vi "SLM Save Frame 640.vi"(4 "Pixel Values":u8[](array[numeric]), 5 "error in (no error)":errorcluster, 6 "Frame Number":u32, 7 "Number of Pixels":u32, 8 "VISA Resource Name":refnum<visa-resource-name>) -> (0 "error out":errorcluster, 3 "dup VISA resource name":refnum<visa-resource-name>)   [LabVIEW 2022 SP3]
panel:
  out "num pixels":u32(graph)
  out "size(s)":i32(graph)
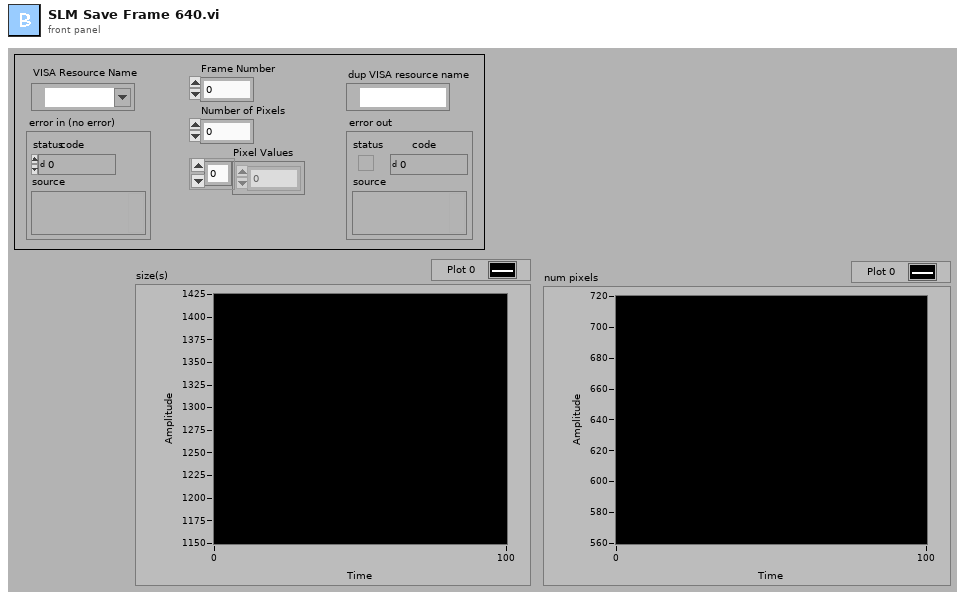
[diagram p1: front panel]
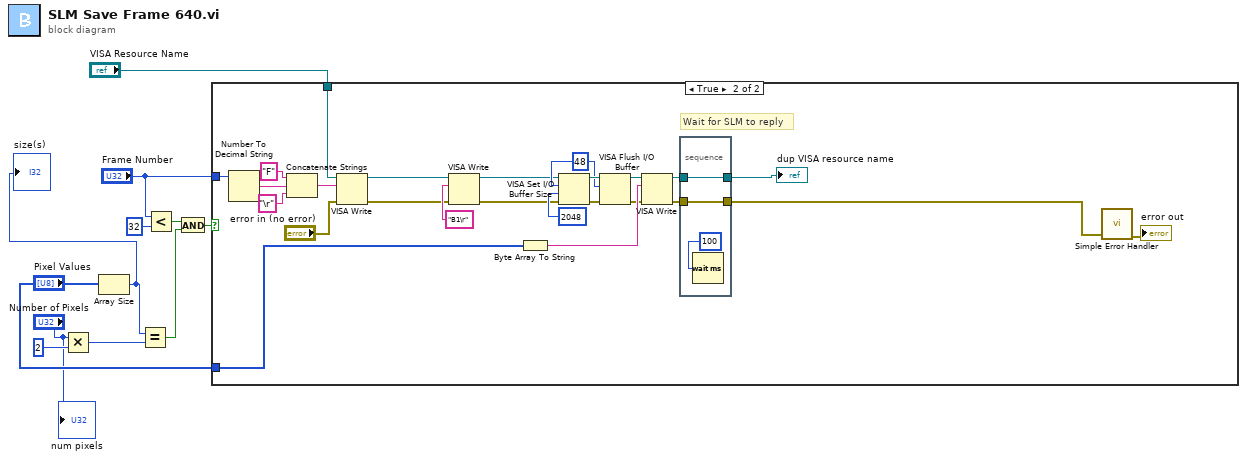
[diagram p0: block diagram]
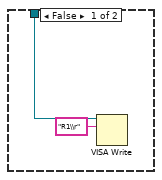
[diagram p2: hidden frame]
diagram:
  n1 = Multiply(x="Number of Pixels", y=2) -> (x*y=w3:u32)
  n2 = Array Size(array="Pixel Values") -> (size(s)=w7:i32)
  "size(s)" <- w7
  n3 = Equal?(x=w7, y=w3) -> (x = y?=w5:bool)
  n4 = Less?(x="Frame Number", y=u8 32) -> (x < y?=w4:bool)
  n5 = And(x=w4, y=w5) -> (x .and. y?=w6:bool)
  n6 = case shown="True" w6 {
    tunnel: "Frame Number" -> [_ w32]
    tunnel: "Pixel Values" -> [_ w29]
    tunnel: "VISA Resource Name" -> [w13 w16]
    frame False {
      n7 = VISA Write(VISA resource name=w13, write buffer="R1\\r") -> ()  [unwired: 1 in, 3 out]
    }
    frame True {
      w21 = u16 48 ("mask (16)")
      # "Wait for SLM to reply"
      n8 = Number To Decimal String(number=w32) -> (decimal integer string=w34:string)  [unwired: 1 in]
      n9 = Concatenate Strings("F" ("Substring"), w34, "\r" ("Substring")) -> (w36:string)
      n10 = VISA Write(VISA resource name=w16, write buffer=w36, error in (no error)="error in (no error)") -> (VISA resource name out=w20:refnum<visa-resource-name>, error out=w19:errorcluster)  [unwired: 1 out]
      n11 = VISA Write(VISA resource name=w20, write buffer="B1\r" ("write buffer (\"\")"), error in (no error)=w19) -> (VISA resource name out=w18:refnum<visa-resource-name>, error out=w17:errorcluster)  [unwired: 1 out]
      n12 = Byte Array To String(unsigned byte array=w29) -> (string=w30:string)
      n13 = VISA Set I/O Buffer Size(VISA resource name=w18, mask (16)=w21, size (4096)=u32 2048 ("size (0)"), error in (no error)=w17) -> (VISA resource name out=w24:refnum<visa-resource-name>, error out=w23:errorcluster)
      n14 = VISA Flush I/O Buffer(VISA resource name=w24, mask (16)=w21, error in (no error)=w23) -> (VISA resource name out=w26:refnum<visa-resource-name>, error out=w25:errorcluster)
      n15 = VISA Write(VISA resource name=w26, write buffer=w30, error in (no error)=w25) -> (VISA resource name out=w28:refnum<visa-resource-name>, error out=w27:errorcluster)  [unwired: 1 out]
      n16 = stacked-sequence {
        tunnel: w28 -> [w40]
        tunnel: [w40] -> w15
        tunnel: w27 -> [w39]
        tunnel: [w39] -> w14
        frame #0 {
          n17 = Wait (ms)(milliseconds to wait=u32 100) -> ()  [unwired: 1 out]
        }
      }
      "dup VISA resource name" <- w15
      n18 = call <vilib>:"Simple Error Handler.vi"("error in (no error)"=w14) -> ("error out"=→"error out":errorcluster)  [unwired: 4 in, 4 out]
    }
  }
  "num pixels" <- "Number of Pixels"
